vi "Write Error.vi"(8 "error in (no error)":errorcluster, 11 "LabVIEW Object":refnum<class>) -> ()   [LabVIEW 2017, in "Integration Test Launcher.lvlib"]
doc: "DO NOT USE THIS ERROR PANEL IN A REAL APPLICATION.\n\nIt is for short-term framework integration testing only. This error panel is a known (intentional) memory leak.\n\n<License>\nCopyright © 2020 Tymphany, LLC | All rights reserved\nwww.Tymphany.com\nHuijun <Huijun.Guo@Tymphany.com>\n</License>"
uses:
  <vilib>/gpm_packages/@cs/example/Integration Test/Integration Test Launcher.lvlib
panel:
  out "Errors and Warnings":string
  # "(A very low-tech singleton logger for framework testing.)"
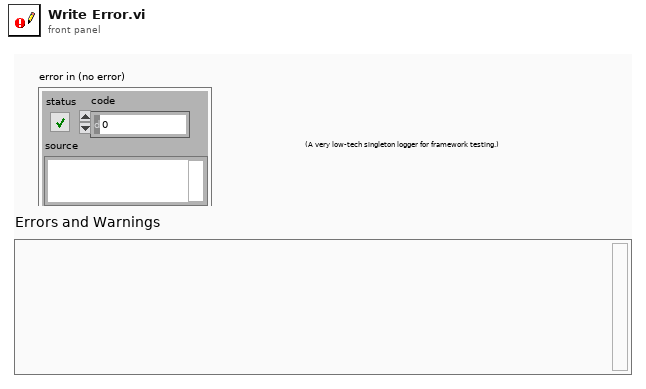
[diagram p1: front panel]
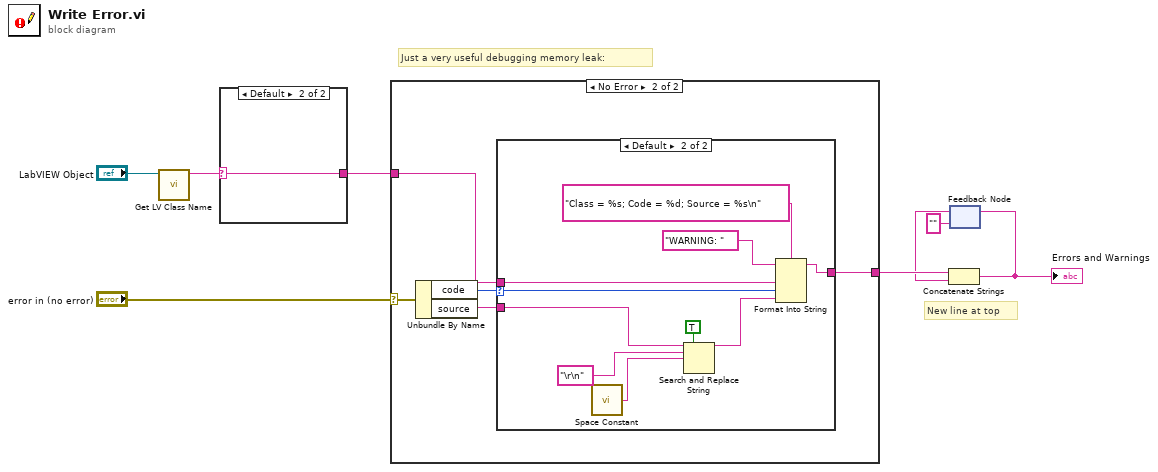
[diagram p0: block diagram]
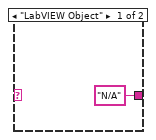
[diagram p2: hidden frame]
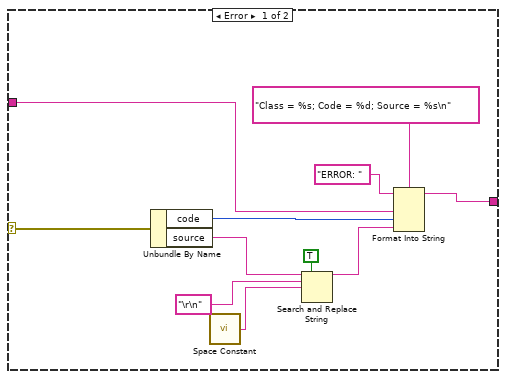
[diagram p3: hidden frame]
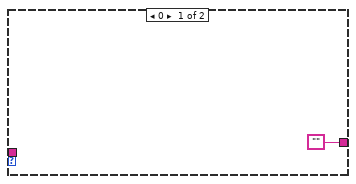
[diagram p4: hidden frame]
diagram:
  # "New line at top"
  # "Just a very useful debugging memory leak:"
  n1 = call <vilib>:"Get LV Class Name.vi"("object"="LabVIEW Object") -> ("class name"=w5:string)  [unwired: 9 in, 1 out]
  n2 = case shown="Default" w5 {
    selector: w5 -> [_ w10]
    tunnel: ["N/A" w10] -> w3
    frame "LabVIEW Object" {
    }
    frame Default {
    }
  }
  n3 = case shown="No Error" "error in (no error)" {
    selector: "error in (no error)" -> [w21 w26]
    tunnel: [w12 w24] -> w8
    tunnel: w3 -> [w11 w22]
    frame Error {
      n4 = Unbundle By Name(w21) -> ("code"=w20:i32, "source"=w19:string)
      n5 = call <vilib>:"Space Constant.vi"() -> ("String"=w17:string)
      n6 = Search and Replace String(replace all?=TRUE ("replace all? (F)"), input string=w19, search string="\r\n", replace string=w17) -> (result string=w15:string)  [unwired: 4 in, 3 out]
      n7 = Format Into String(format string="Class = %s; Code = %d; Source = %s\n", initial string="ERROR: ", w11, w20, w15) -> (resulting string=w12:string)  [unwired: 1 in, 1 out]
    }
    frame No Error {
      n8 = Unbundle By Name(w26) -> ("code"=w23:i32, "source"=w25:string)
      n9 = case shown="Default" w23 {
        selector: w23 -> [_ w29]
        tunnel: w25 -> [_ w37]
        tunnel: ["" w30] -> w24
        tunnel: w22 -> [_ w28]
        frame 0 {
        }
        frame Default {
          n10 = call <vilib>:"Space Constant.vi"() -> ("String"=w35:string)
          n11 = Search and Replace String(replace all?=TRUE ("replace all? (F)"), input string=w37, search string="\r\n", replace string=w35) -> (result string=w33:string)  [unwired: 4 in, 3 out]
          n12 = Format Into String(format string="Class = %s; Code = %d; Source = %s\n", initial string="WARNING: ", w28, w29, w33) -> (resulting string=w30:string)  [unwired: 1 in, 1 out]
        }
      }
    }
  }
  n13 = feedback #1("") -> (w7:string)
  n14 = Concatenate Strings(w8, w7) -> (w6:string)
  "Errors and Warnings" <- w6
  n15 = feedback-in #1(w6) -> ()
